vi "Stop VIs.vi"   [LabVIEW 2014]
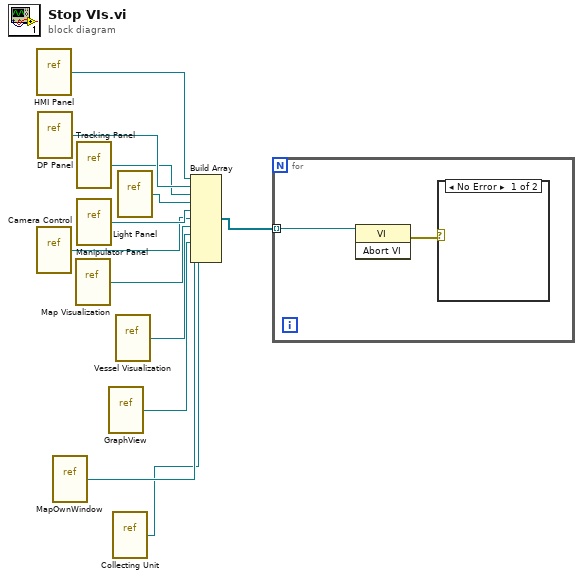
[diagram p0: block diagram]
diagram:
  n1 = vi-ref "HMI Panel.vi"() -> (w4:refnum<vi>)
  n2 = vi-ref "Camera Control.vi"() -> (w8:refnum<vi>)
  n3 = vi-ref "DP Panel.vi"() -> (w12:refnum<vi>)
  n4 = vi-ref "MapOwnWindow.vi"() -> (w2:refnum<vi>)
  n5 = vi-ref "Map Visualization.vi"() -> (w7:refnum<vi>)
  n6 = vi-ref "Tracking Panel.vi"() -> (w11:refnum<vi>)
  n7 = vi-ref "Manipulator Panel.vi"() -> (w9:refnum<vi>)
  n8 = vi-ref "GraphView.vi"() -> (w3:refnum<vi>)
  n9 = vi-ref "Collecting Unit.vi"() -> (w1:refnum<vi>)
  n10 = vi-ref "Vessel Visualization.vi"() -> (w6:refnum<vi>)
  n11 = vi-ref "Light Panel.vi"() -> (w10:refnum<vi>)
  n12 = Build Array(w4, w12, w11, w10, w9, w8, w7, w6, w3, w2, w1) -> (w5:refnum<vi>[])
  n13 = for {
    tunnel: w5 -> [w14] mode=indexing
    n14 = invoke class="VI" method="Abort VI"(reference=w14) -> (error out=w13:errorcluster)  [unwired: 2 in, 2 out]
    n15 = case shown="No Error" w13 {
      frame No Error {
      }
      frame Error {
      }
    }
  }
